vi "SelectMarker.vi"(0 "VISA IN":refnum<visa-resource-name>, 1 "Marker":T1(ring), 5 "error in":errorcluster, 7 "Channel":i32=1, 9 "ON-OFF":bool) -> (14 "VISA Out":refnum<visa-resource-name>, 19 "error out":errorcluster)   [LabVIEW 2018, in "PNA-X.lvlib"]
uses:
  PNA-X.lvlib
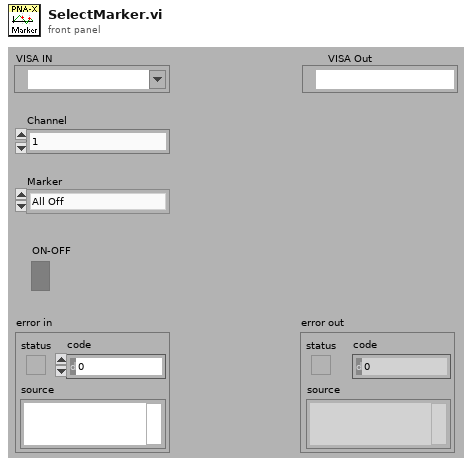
[diagram p1: front panel]
types:
  T1 = enum16{"All Off", "1", "2", "3", "4", "5", "6", "7", "8", "9", "Reference"}
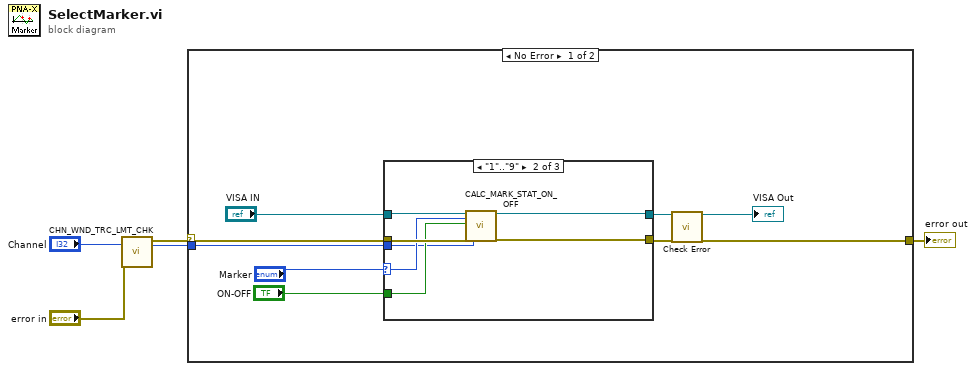
[diagram p0: block diagram]
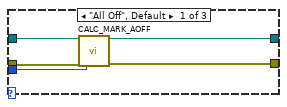
[diagram p2: hidden frame]
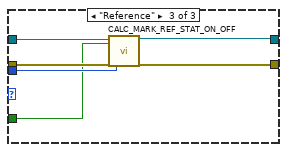
[diagram p3: hidden frame]
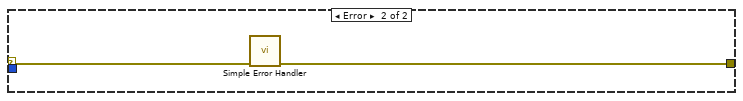
[diagram p4: hidden frame]
diagram:
  n1 = call "CHN_WND_TRC_LMT_CHK.vi"("Channel"="Channel", "error in"="error in") -> ("error out"=w2:errorcluster, "Channel"=w1:i32)  [unwired: 13 in, 3 out]
  n2 = case shown="No Error" w2 {
    selector: w2 -> [w12 w34]
    tunnel: [w14 w33] -> w4
    tunnel: w1 -> [w10 _]
    frame No Error {
      n3 = case shown="\"1\"..\"9\"" "Marker" {
        selector: "Marker" -> [_ w24 _]
        tunnel: w12 -> [w19 w26 w32]
        tunnel: [w18 w21 w29] -> w6
        tunnel: w10 -> [w17 w22 w28]
        tunnel: "VISA IN" -> [w16 w25 w31]
        tunnel: [w15 w20 w30] -> w7
        tunnel: "ON-OFF" -> [_ w23 w27]
        frame "All Off", Default {
          n4 = call "CALC_MARK_AOFF.vi"("VISA IN"=w16, "error in"=w19, "Channel"=w17) -> ("VISA Out"=w15:refnum<visa-resource-name>, "error out"=w18:errorcluster)  [unwired: 15 in]
        }
        frame "1".."9" {
          n5 = call "CALC_MARK_STAT_ON_OFF.vi"("VISA IN"=w25, "Marker number"=w24, "Marker ON/OFF"=w23, "error in"=w26, "Channel"=w22) -> ("VISA Out"=w20:refnum<visa-resource-name>, "error out"=w21:errorcluster)  [unwired: 13 in]
        }
        frame "Reference" {
          n6 = call "CALC_MARK_REF_STAT_ON_OFF.vi"("VISA IN"=w31, "Reference Marker ON/OFF"=w27, "error in"=w32, "Channel"=w28) -> ("VISA Out"=w30:refnum<visa-resource-name>, "error out"=w29:errorcluster)  [unwired: 14 in]
        }
      }
      n7 = call "Check Error.vi"("VISA Resource Name"=w7, "error in (no error)"=w6) -> ("dup VISA session"=→"VISA Out":refnum<visa-resource-name>, "error out"=w14:errorcluster)  [unwired: 16 in]
    }
    frame Error {
      n8 = call <vilib>:"Simple Error Handler.vi"("error in (no error)"=w34) -> ("error out"=w33:errorcluster)  [unwired: 4 in, 4 out]
    }
  }
  "error out" <- w4
